vi "autonomous.vi"() -> ()   [LabVIEW 2012, in "MainProject.lvrbt"]
uses:
  Drivers/AutoDriverControl.ctl
  <vilib>/NXT/HiTechnic/HiTechnic Controls/HiTechnic Port.ctl
  <vilib>/NXT/Block Support/NXT_InputPort.ctl
  <vilib>/NXT/Hardware/Plugins/Tetrix DC Motor/TetrixDCMotorAddress.ctl
  <vilib>/NXT/Hardware/Plugins/Tetrix 180 deg Servo/Tetrix180ServoAddress.ctl
  FTC 2012 - 2013/Controls/SpeedControl.ctl
  Drivers/LineCountColorCtl.ctl
  <vilib>/NXT/NXTIO Xnodes/NXTIONodeSubVIs/TETRIX IO Check Battery.vi
  <vilib>/NXT/Dual Mode Library/Waits/Wait_Num(msec).vi
  <vilib>/NXT/NXTIO Xnodes/NXTIONodeSubVIs/TETRIX IO Move Servos.vi
  <vilib>/NXT/NXTIO Xnodes/NXTIONodeSubVIs/TETRIX IO Stop DC Motors.vi
  <vilib>/NXT/Dual Mode Library/Waits/Wait_Num.vi
  <vilib>/NXT/Dual Mode Library/Sound/Tone.vi
  <vilib>/NXT/Subs/LVHSConnector.ctl
  <vilib>/NXT/NXTIO Xnodes/AddressXNode/NXTIOAddress.xnode
  MainProject.lvrbt
  <vilib>/NXT/NXTIO Xnodes/NXTIOXNode/NXTIO.xnode
  <vilib>/NXT/LegoClasses/BrickReference/BrickReference.lvclass
panel:
  out "Enabled":bool
  out "Line Color":string="Black"
  out "Sector (0-9)":i16
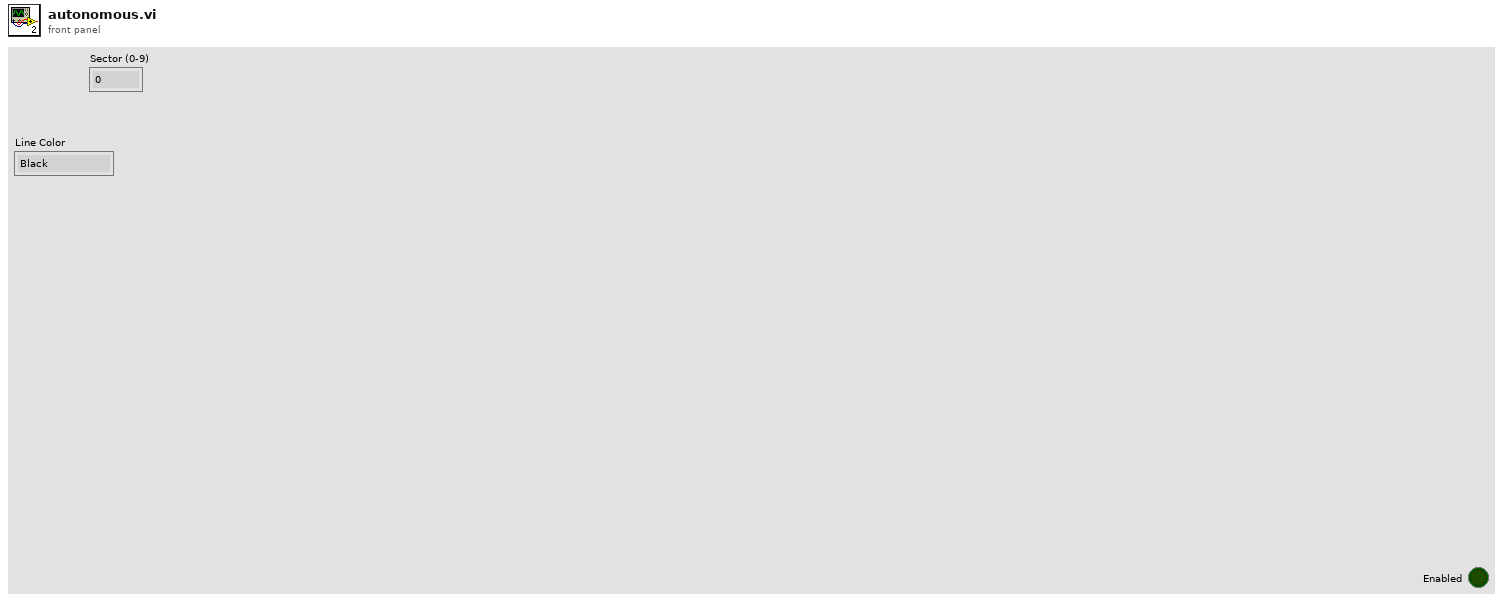
[diagram p1: front panel]
types:
  T1 = typedef "HiTechnic Port.ctl" = cluster{"Port":T2, "MUX Port":u8}
  T2 = typedef "NXT_InputPort.ctl" = u8
  T3 = typedef "AutoDriverControl.ctl" = enum16{"Init", "Forward", "Reverse", "Left", "Right", "Brake"}
  T4 = typedef "TetrixDCMotorAddress.ctl" = i16
  T5 = typedef "LVHSConnector.ctl" = refnum<class "BrickReference.lvclass">
  T6 = typedef "AutoControl3.ctl" = enum16{"FindIRBasket", "DropBLK", "DrvToEndOfBaskets", "DrvAroundBaskets", "AlignWithRamp", "ParkOnRamp", "Stop"}
  T7 = typedef "Tetrix180ServoAddress.ctl" = i16
  T8 = cluster{"Tetrix180Servo":T7, "Tetrix180Servo":T7, "Tetrix180Servo":T7, "Tetrix180Servo":T7}
  T9 = typedef "LineCountColorCtl.ctl" = enum16{"Init/Reset", "Check"}
  T10 = typedef "SpeedControl.ctl" = enum16{"Fast", "Medium", "Slow"}
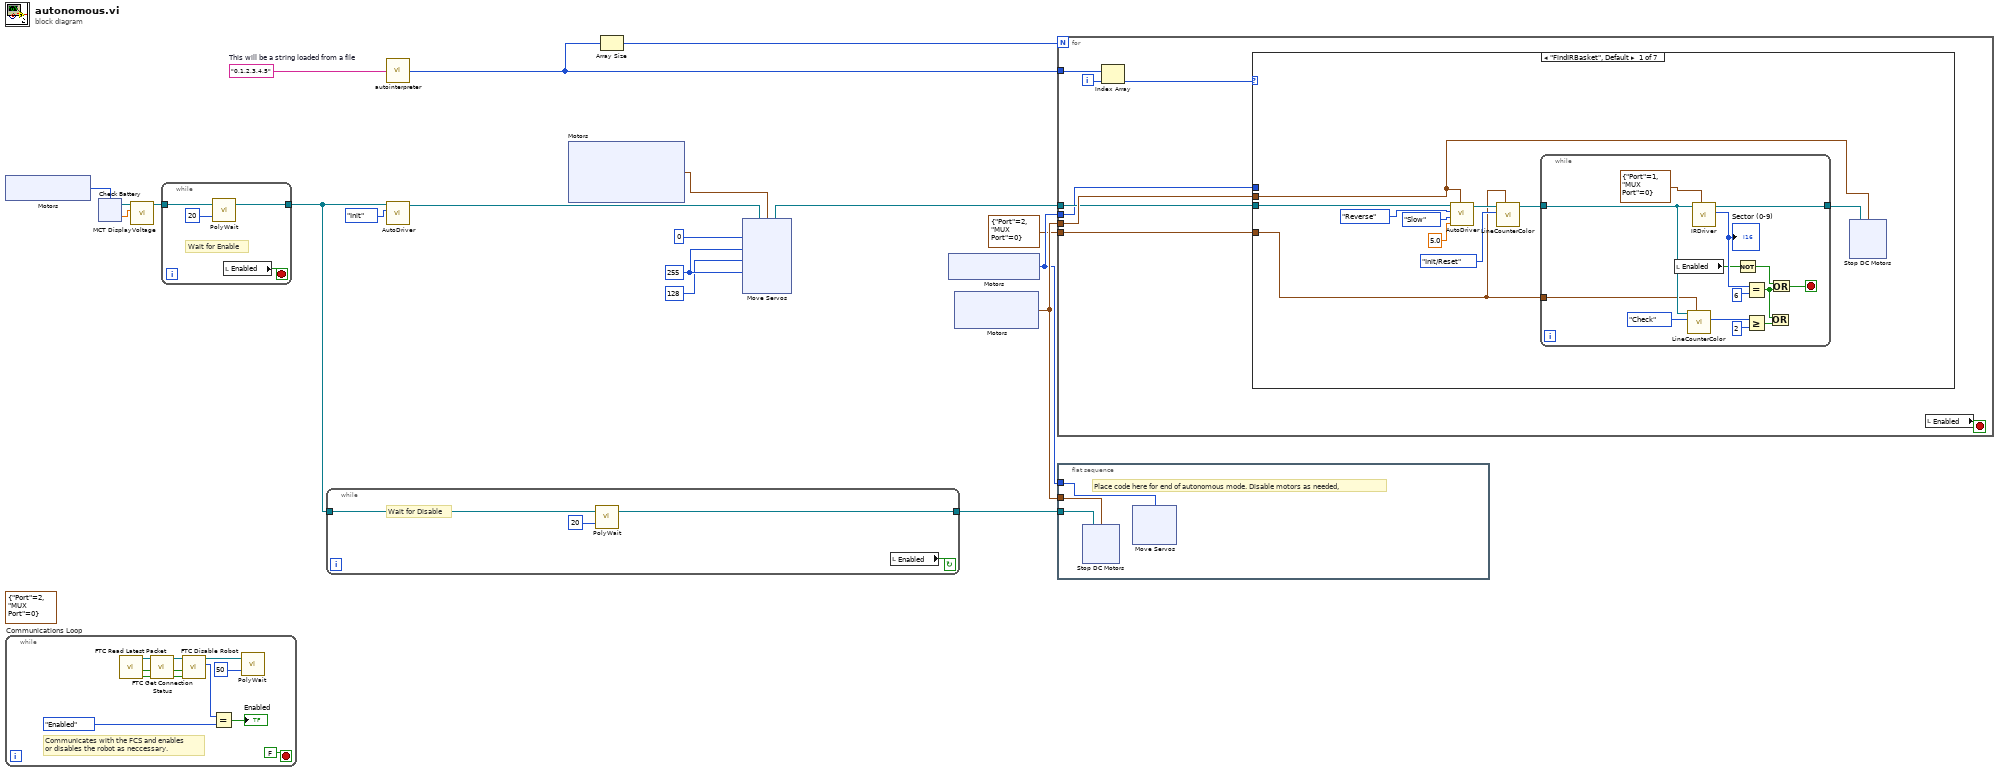
[diagram p0: block diagram]
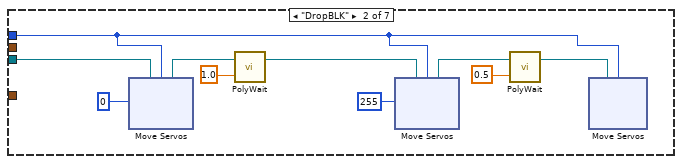
[diagram p2: hidden frame]
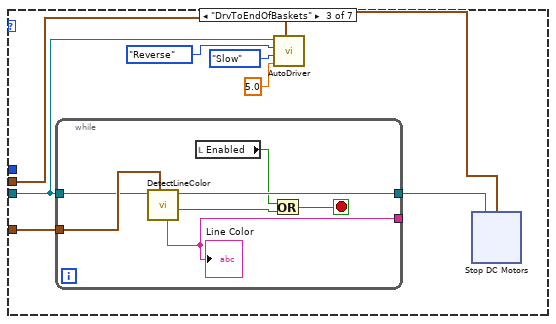
[diagram p3: hidden frame]
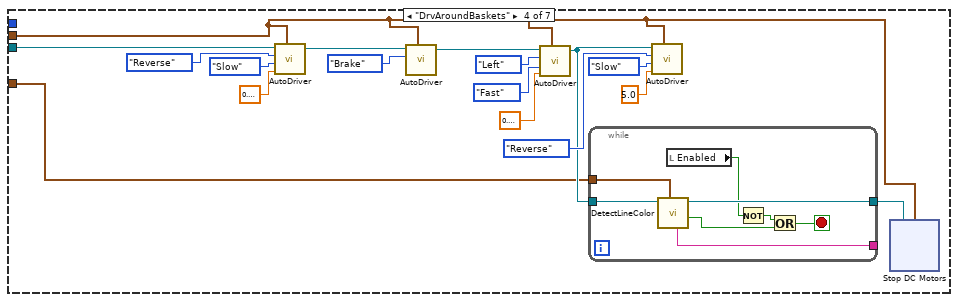
[diagram p4: hidden frame]
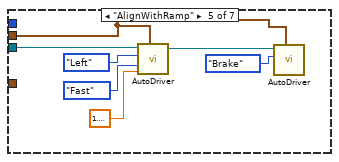
[diagram p5: hidden frame]
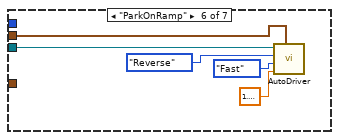
[diagram p6: hidden frame]
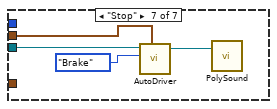
[diagram p7: hidden frame]
diagram:
  w9 = u8 255 ("Position 2")
  (unwired) T1 {"Port"=2, "MUX Port"=0} ("Port/MUX")
  w19 = "0,1,2,3,4,5"  # This will be a string loaded from a file
  n1 = xnode "Motors"() -> ("Motor"=w13:T4)
  n2 = while "Communications Loop" {
    stop <- FALSE stop-if-true
    # "Communicates with the FCS and enables \nor disables the robot as neccessary."
    n3 = call <vilib>:"FTC Read Latest Packet.vi"() -> ("Packet Received?"=w29:bool, "Stopped?"=w28:bool, "NXT"=w31:T5)  [unwired: 6 in, 3 out]
    n4 = call <vilib>:"FTC Get Connection Status.vi"("Packet Received?"=w29, "Stopped?"=w28, "NXT"=w31) -> ("Online?"=w21:bool, "Stopped?"=w22:bool, "NXT"=w30:T5)  [unwired: 5 in]
    n5 = call <vilib>:"FTC Disable Robot.vi"("Online?"=w21, "Stopped?"=w22, "NXT"=w30) -> ("Enabled?"=w24:enum16{"Disabled", "Enabled"}, "NXT"=w26:T5)  [unwired: 3 in]
    n6 = Equal?(x=w24, y=enum16{"Disabled", "Enabled"}."Enabled") -> (x = y?=→"Enabled":bool)
    n7 = call-poly <vilib>:"PolyWait.vi"("Time (100 msec)"=u32 50 ("Time (msec)"), "NXT"=w26) -> ()  [unwired: 2 in, 1 out]
  }
  n8 = xnode "Check Battery"("Motors"=w13) -> ("Voltage 1"=w15:sgl, "NXT"=w16:T5)  [unwired: 1 in]
  n9 = call <vilib>:"MCT DisplayVoltage.vi"("Motor Voltage"=w15, "NXT"=w16) -> ("NXT"=w14:T5)  [unwired: 9 in]
  n10 = while {
    tunnel: [w34] -> w3
    tunnel: w14 -> [w33]
    stop <- w32 stop-if-true
    # "Wait for Enable"
    n11 = call-poly <vilib>:"PolyWait.vi"("Time (100 msec)"=u32 20 ("Time (msec)"), "NXT"=w33) -> ("NXT"=w34:T5)  [unwired: 2 in]
    n12 = local read "Enabled"() -> (w32:bool)
  }
  n13 = while {
    tunnel: w3 -> [w38]
    tunnel: [w36] -> w12
    stop <- w37 continue-if-true
    # "Wait for Disable"
    n14 = call-poly <vilib>:"PolyWait.vi"("Time (100 msec)"=u32 20 ("Time (msec)"), "NXT"=w38) -> ("NXT"=w36:T5)  [unwired: 2 in]
    n15 = local read "Enabled"() -> (w37:bool)
  }
  n16 = call "autointerpreter.vi"("String"=w19) -> ("Array"=w17:T6[])
  n17 = call "AutoDriver.vi"("NXT In"=w3, "Direction"=AutoDriverControl."Init") -> ("NXT Out"=w5:T5)  [unwired: 6 in]
  n18 = xnode "Motors"() -> ("Motor"=w4:T8)
  n19 = Array Size(array=w17) -> (size(s)=w18:i32)
  n20 = xnode "Move Servos"("Position 4"=w9, "Position 3"=u8 128 ("Position 5"), "Position 2"=w9, "Position 1"=u8 0, "Servos"=w4, "NXT"=w5) -> ("NXT"=w2:T5)
  n21 = xnode "Motors"() -> ("Motor"=w10:T7)
  n22 = xnode "Motors"() -> ("Motor"=w11:cluster{"TetrixDCMotor":T4, "TetrixDCMotor":T4})
  n23 = for {
    N: w18 -> [_]
    tunnel: w17 -> [w47]
    tunnel: w11 -> [w45]
    tunnel: w2 -> [w44]
    tunnel: w10 -> [w42]
    tunnel: T1 {"Port"=2, "MUX Port"=0} ("Port/MUX") -> [w41]
    i -> [w46]
    stop <- w40 stop-if-true
    n24 = Index Array(array=w47, index=w46) -> (element=w43:T6)
    n25 = case shown="\"FindIRBasket\", Default" w43 {
      tunnel: w45 -> [w49 _ w110 w131 w163 w170 w175]
      tunnel: w44 -> [w50 w79 w111 w133 w164 w171 w176]
      tunnel: w42 -> [_ w80 _ _ _ _ _]
      tunnel: w41 -> [w48 _ w112 w132 _ _ _]
      frame "FindIRBasket", Default {
        n26 = call "AutoDriver.vi"("NXT In"=w50, "Motors"=w49, "Direction"=AutoDriverControl."Reverse", "Speed"=SpeedControl."Slow", "Time (1 sec)"=sgl 5.0) -> ("NXT Out"=w51:T5)  [unwired: 3 in]
        n27 = call "LineCounterColor.vi"("Port/MUX"=w48, "Enum"=LineCountColorCtl."Init/Reset", "NXT In"=w51) -> ("NXT Out"=w53:T5)  [unwired: 7 in, 1 out]
        n28 = while {
          tunnel: w53 -> [w67]
          tunnel: [w73] -> w54
          tunnel: w48 -> [w66]
          stop <- w71 stop-if-true
          n29 = local read "Enabled"() -> (w65:bool)
          n30 = call "LineCounterColor.vi"("Port/MUX"=w66, "Enum"=LineCountColorCtl."Check", "NXT In"=w67) -> ("Numeric"=w69:i16)  [unwired: 7 in, 1 out]
          n31 = call "IRDriver.vi"("Port"=T1 {"Port"=1, "MUX Port"=0}, "NXT In"=w67) -> ("Sector (0-9)"=w77:i16, "NXT Out"=w73:T5)  [unwired: 8 in]
          "Sector (0-9)" <- w77
          n32 = Not(x=w65) -> (.not. x?=w70:bool)
          n33 = Equal?(x=w77, y=i16 6) -> (x = y?=w68:bool)
          n34 = Greater Or Equal?(x=w69, y=i16 2) -> (x >= y?=w74:bool)
          n35 = Or(x=w68, y=w74) -> ()  [unwired: 1 out]
          n36 = Or(x=w70, y=w68) -> (x .or. y?=w71:bool)
        }
        n37 = xnode "Stop DC Motors"("Motors"=w49, "NXT"=w54) -> ()  [unwired: 1 out]
      }
      frame "DropBLK" {
        n38 = xnode "Move Servos"("Position 1"=u8 0, "Servos"=w80, "NXT"=w79) -> ("NXT"=w81:T5)
        n39 = call-poly <vilib>:"PolyWait.vi"("Time (1 sec)"=sgl 1.0, "NXT"=w81) -> ("NXT"=w87:T5)  [unwired: 2 in]
        n40 = xnode "Move Servos"("Position 1"=u8 255, "Servos"=w80, "NXT"=w87) -> ("NXT"=w86:T5)
        n41 = call-poly <vilib>:"PolyWait.vi"("Time (1 sec)"=sgl 0.5, "NXT"=w86) -> ("NXT"=w83:T5)  [unwired: 2 in]
        n42 = xnode "Move Servos"("Servos"=w80, "NXT"=w83) -> ()  [unwired: 1 in, 1 out]
      }
      frame "DrvToEndOfBaskets" {
        n43 = while {
          tunnel: [w130] -> w113
          tunnel: [w129] -> _
          tunnel: w112 -> [w128]
          tunnel: w111 -> [w127]
          stop <- w125 stop-if-true
          n44 = call "DetectLineColor.vi"("Port/MUX"=w128, "NXT In"=w127) -> ("Detected Line?"=w126:bool, "NXT Out"=w130:T5, "Color"=w129:string)  [unwired: 7 in]
          "Line Color" <- w129
          n45 = local read "Enabled"() -> (w124:bool)
          n46 = Or(x=w124, y=w126) -> (x .or. y?=w125:bool)
        }
        n47 = call "AutoDriver.vi"("NXT In"=w111, "Motors"=w110, "Direction"=AutoDriverControl."Reverse", "Speed"=SpeedControl."Slow", "Time (1 sec)"=sgl 5.0) -> ()  [unwired: 3 in, 1 out]
        n48 = xnode "Stop DC Motors"("Motors"=w110, "NXT"=w113) -> ()  [unwired: 1 out]
      }
      frame "DrvAroundBaskets" {
        n49 = call "AutoDriver.vi"("NXT In"=w133, "Motors"=w131, "Direction"=AutoDriverControl."Reverse", "Speed"=SpeedControl."Slow", "Time (1 sec)"=sgl 0.3) -> ("NXT Out"=w141:T5)  [unwired: 3 in]
        n50 = call "AutoDriver.vi"("NXT In"=w141, "Motors"=w131, "Direction"=AutoDriverControl."Brake") -> ("NXT Out"=w140:T5)  [unwired: 5 in]
        n51 = call "AutoDriver.vi"("NXT In"=w140, "Motors"=w131, "Direction"=AutoDriverControl."Left", "Speed"=SpeedControl."Fast", "Time (1 sec)"=sgl 0.8) -> ("NXT Out"=w135:T5)  [unwired: 3 in]
        n52 = while {
          tunnel: [w162] -> _
          tunnel: [w161] -> w134
          tunnel: w135 -> [w157]
          tunnel: w132 -> [w156]
          stop <- w159 stop-if-true
          n53 = call "DetectLineColor.vi"("Port/MUX"=w156, "NXT In"=w157) -> ("Detected Line?"=w160:bool, "NXT Out"=w161:T5, "Color"=w162:string)  [unwired: 7 in]
          n54 = local read "Enabled"() -> (w155:bool)
          n55 = Not(x=w155) -> (.not. x?=w158:bool)
          n56 = Or(x=w158, y=w160) -> (x .or. y?=w159:bool)
        }
        n57 = call "AutoDriver.vi"("NXT In"=w135, "Motors"=w131, "Direction"=AutoDriverControl."Reverse", "Speed"=SpeedControl."Slow", "Time (1 sec)"=sgl 5.0) -> ()  [unwired: 3 in, 1 out]
        n58 = xnode "Stop DC Motors"("Motors"=w131, "NXT"=w134) -> ()  [unwired: 1 out]
      }
      frame "AlignWithRamp" {
        n59 = call "AutoDriver.vi"("NXT In"=w164, "Motors"=w163, "Direction"=AutoDriverControl."Left", "Speed"=SpeedControl."Fast", "Time (1 sec)"=sgl 1.1) -> ("NXT Out"=w166:T5)  [unwired: 3 in]
        n60 = call "AutoDriver.vi"("NXT In"=w166, "Motors"=w163, "Direction"=AutoDriverControl."Brake") -> ()  [unwired: 5 in, 1 out]
      }
      frame "ParkOnRamp" {
        n61 = call "AutoDriver.vi"("NXT In"=w171, "Motors"=w170, "Direction"=AutoDriverControl."Reverse", "Speed"=SpeedControl."Fast", "Time (1 sec)"=sgl 1.3) -> ()  [unwired: 3 in, 1 out]
      }
      frame "Stop" {
        n62 = call "AutoDriver.vi"("NXT In"=w176, "Motors"=w175, "Direction"=AutoDriverControl."Brake") -> ("NXT Out"=w177:T5)  [unwired: 5 in]
        n63 = call-poly <vilib>:"PolySound.vi"("NXT"=w177) -> ()  [unwired: 3 in, 1 out]
      }
    }
    n64 = local read "Enabled"() -> (w40:bool)
  }
  n65 = flat-sequence {
    tunnel: w11 -> [w180]
    tunnel: w10 -> [w181]
    tunnel: w12 -> [w179]
    frame #0 {
      # "Place code here for end of autonomous mode. Disable motors as needed,"
      n66 = xnode "Stop DC Motors"("Motors"=w180, "NXT"=w179) -> ()  [unwired: 1 out]
      n67 = xnode "Move Servos"("Servos"=w181) -> ()  [unwired: 2 in, 1 out]
    }
  }
